vi "peek.vi"(6 "timeout (25000ms)":i32=25000, 8 "error in (no error)":errorcluster, 10 "parameter name":string, 11 "daemon reference in":refnum<k5>) -> (0 "error out":errorcluster, 2 "value":i32, 3 "daemon reference out":refnum<k5>, 5 "command out":string="random")   [LabVIEW 2017]
doc: "<b>Command: </b>\"peek\"\n\n<b>Description: </b>This command peeks at a variable stored in memory on the target.\n\n<b>Parameters: </b> \n\n 1. Name of variable to peek\n\n<b>Note: </b>This command will only work on DEV builds of the target and as long as the relevant firmware json file has been loaded using \"load_firmware_json\" command.\n____________________________________________\nDIPC 692 Daemon API 10.0.0.1\nSam Tee - Dyson Technology Ltd\nCopyright (c) 2024, Dyson Technology Ltd"
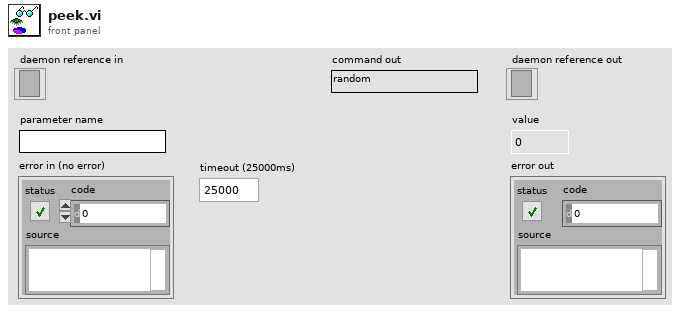
[diagram p1: front panel]
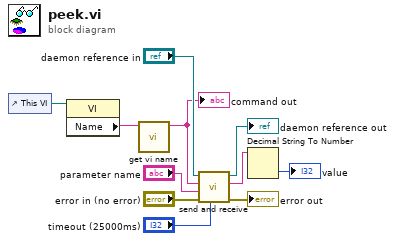
[diagram p0: block diagram]
diagram:
  n1 = control-ref of="This VI"() -> (w6:refnum<vi>)
  n2 = property class="VI"(reference=w6) -> ("Name"=w4:string)  [unwired: 1 in, 2 out]
  n3 = call "get vi name.vi"("library.lvlib:name.vi"=w4) -> ("vi name"=w3:string)  [unwired: 10 in]
  "command out" <- w3
  n4 = call "send and receive.vi"("timeout (25000ms)"="timeout (25000ms)", "error in (no error)"="error in (no error)", "data"="parameter name", "command"=w3, "daemon reference in"="daemon reference in") -> ("error out"=→"error out":errorcluster, "response"=w2:string, "daemon reference out"=→"daemon reference out":refnum<k5>)  [unwired: 4 in]
  n5 = Decimal String To Number(string=w2) -> (number=→"value":i32)  [unwired: 2 in, 1 out]
